vi "Read Repeat_.vi"(8 "error in (no error)":errorcluster, 11 "DIO in":refnum<class "DIO.lvclass">) -> (0 "error out":errorcluster, 2 "Repeat?":bool, 3 "DIO out":refnum<class "DIO.lvclass">)   [LabVIEW 2015, in "DIO.lvclass"]
uses:
  DIO.lvclass
  DIO.lvclass/DIO.ctl
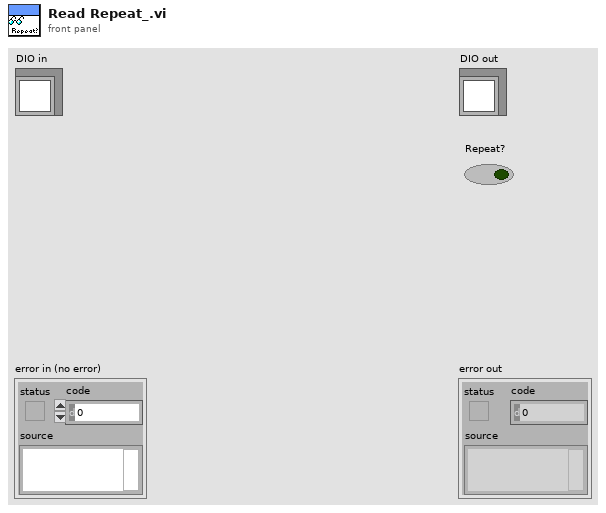
[diagram p1: front panel]
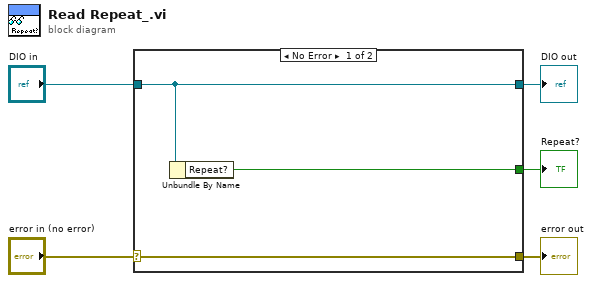
[diagram p0: block diagram]
diagram:
  n1 = case shown="No Error" "error in (no error)" {
    selector: "error in (no error)" -> [w8 w9]
    tunnel: [w8 w9] -> w4
    tunnel: [w7 w10] -> w2
    tunnel: "DIO in" -> [w7 w10]
    tunnel: [w6 _] -> w1
    frame No Error {
      n2 = Unbundle By Name(w7) -> ("Repeat?"=w6:bool)
    }
    frame Error {
    }
  }
  "error out" <- w4
  "DIO out" <- w2
  "Repeat?" <- w1
